vi "Handle Result.vi"(8 "error in (no error)":errorcluster, 10 "Result":T1={"Name"="", "Description"="", "Status"=enum."Passed", "Result Type"=enum."Test Suite", "Execution Time"=0.0, "Data"={"Expected"=variant, "Actual"=variant, "Delta"=variant}}, 11 "XML Report In":refnum<class "XML Report.lvclass">) -> (0 "error out":errorcluster, 3 "XML Report Out":refnum<class "XML Report.lvclass">)   [LabVIEW 2020, in "XML Report.lvclass"]
uses:
  XML Report.lvclass
  Core/Result/Result.ctl
  Core/Result/Status.ctl
  Core/Result/Type.ctl
  Case Result.ctl
  XML Report.lvclass/XML Report.ctl
  <vilib>/Utility/miscctls.llb/LVMapReplaceAction.ctl
  Core/Result/Result.lvlib
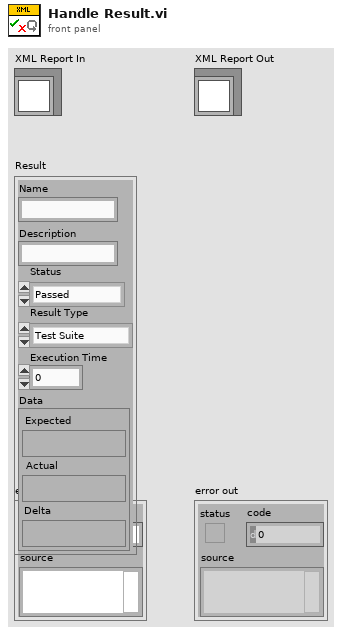
[diagram p1: front panel]
types:
  T1 = typedef "Result.lvlib/Result.ctl" = cluster{"Name":string, "Description":string, "Status":T2, "Result Type":T3, "Execution Time":dbl, "Data":cluster{"Expected":variant, "Actual":variant, "Delta":variant}}
  T2 = typedef "Result.lvlib/Status.ctl" = enum16{"", "Passed", "Failed", "Error", "Skipped", "Setup Error", "Broken", "Teardown Error"}
  T3 = typedef "Result.lvlib/Type.ctl" = enum16{"Test Case", "Test Suite", "Test Run", "Pass", "Fail", "Skip", "Pass if", "Fail if", "Pass if Error", "Fail if Error", "Pass if Equal", "Fail if Equal"}
  T4 = typedef "XML Report.lvclass/Case Result.ctl" = cluster{"Name":string, "Assertions":i32, "Classname":string, "Status":T2, "Time":dbl}
  T5 = typedef "LVMapReplaceAction.ctl" = enum32{"Modify Entry only if found", "Add or Modify Entry", "Delete Entry"}
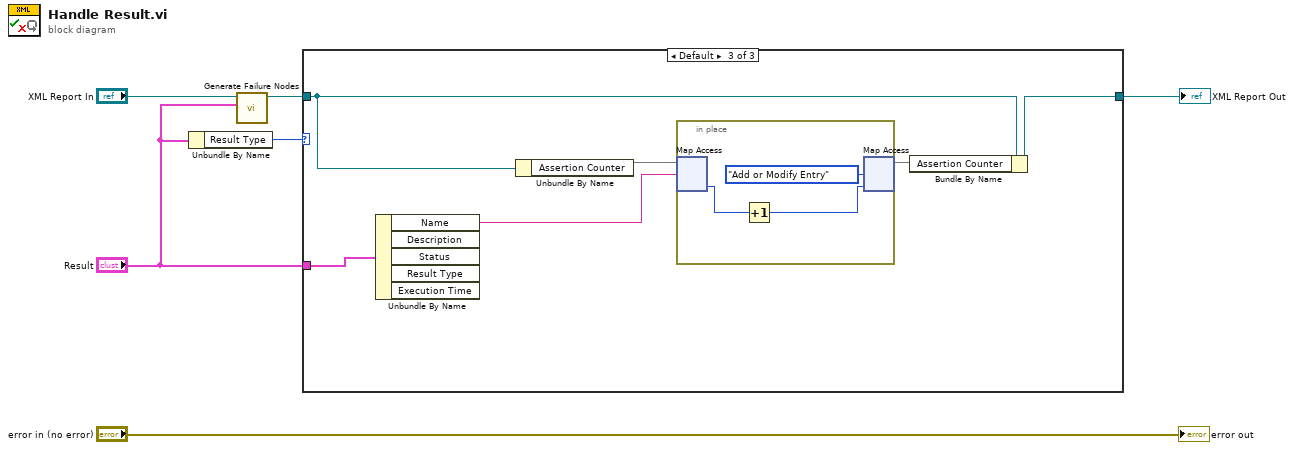
[diagram p0: block diagram]
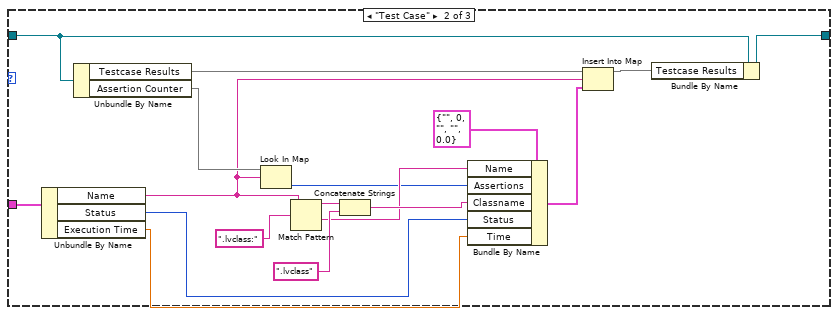
[diagram p3: hidden frame]
diagram:
  n1 = Unbundle By Name("Result") -> ("Result Type"=w4:T3)
  n2 = call "Generate Failure Nodes.vi"("Result"="Result", "XML Report in"="XML Report In") -> ("XML Report out"=w2:refnum<class "XML Report.lvclass">)  [unwired: 9 in]
  n3 = case shown="Default" w4 {
    tunnel: w2 -> [w7 w21 w26]
    tunnel: [w7 w20 w30] -> w5
    tunnel: "Result" -> [_ w24 w25]
    frame "Test Run" {
    }
    frame "Test Case" {
      n4 = Unbundle By Name(w24) -> ("Name"=w11:string, "Status"=w9:T2, "Execution Time"=w8:dbl)
      n5 = Unbundle By Name(w21) -> ("Testcase Results"=w19:map{string, T4}, "Assertion Counter"=w12:map{string, i32})
      n6 = Look In Map(map=w12, key=w11) -> (value=w10:i32)  [unwired: 1 in, 1 out]
      n7 = Match Pattern(string=w11, regular expression=".lvclass:") -> (before substring=w22:string, after substring=w13:string)  [unwired: 1 in, 2 out]
      n8 = Concatenate Strings(w22, ".lvclass" ("string")) -> (w14:string)
      n9 = Bundle By Name(cluster=T4 {"Name"="", "Assertions"=0, "Classname"="", "Status"=enum."", "Time"=0.0} ("value"), "Name"=w13, "Assertions"=w10, "Classname"=w14, "Status"=w9, "Time"=w8) -> (w16:T4)
      n10 = Insert Into Map(map in=w19, key=w11, value=w16) -> (map out=w18:map{string, T4})  [unwired: 2 out]
      n11 = Bundle By Name(cluster=w21, "Testcase Results"=w18) -> (w20:refnum<class "XML Report.lvclass">)
    }
    frame Default {
      n12 = Unbundle By Name(w25) -> ("Name"=w27:string)  [unwired: 4 out]
      n13 = Unbundle By Name(w26) -> ("Assertion Counter"=w29:map{string, i32})
      n14 = in-place {
        n15 = in-place-map #1(w29, w27) -> (w32:i32)  [unwired: 1 in, 1 out]
        n16 = Increment(x=w32) -> (x+1=w31:i32)
        n17 = in-place-map #1(w31, LVMapReplaceAction."Add or Modify Entry" ("action")) -> (w28:map{string, i32})  [unwired: 2 out]
      }
      n18 = Bundle By Name(cluster=w26, "Assertion Counter"=w28) -> (w30:refnum<class "XML Report.lvclass">)
    }
  }
  "XML Report Out" <- w5
  "error out" <- "error in (no error)"
